vi "FindVideoDevices.vi"(8 "error in (no error)":errorcluster, 11 "Path to FFMPEG":path=path "C:/Program Files/FFMpeg/bin/ffmpeg.exe") -> (0 "error out":errorcluster, 3 "Video Devices":string[](array[string]))   [LabVIEW 2024]
uses:
  <userlib>/_OpenG.lib/array/array.llb/Conditional Auto-Indexing Tunnel (String)__ogtk.vi
  <vilib>/regexp/Match Regular Expression.xnode
  <userlib>/_OpenG.lib/string/string.llb/openg_string.lvlib
  <userlib>/_OpenG.lib/array/array.llb/openg_array.lvlib
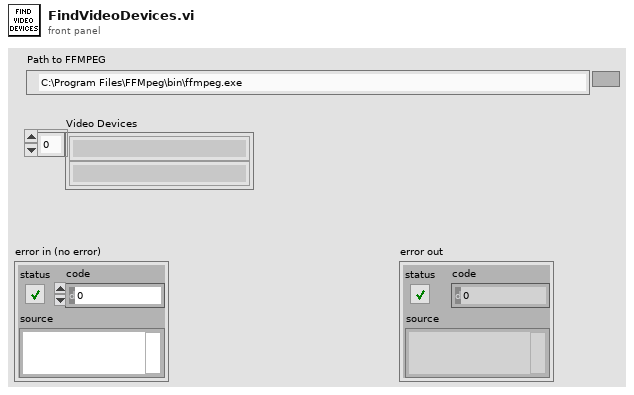
[diagram p1: front panel]
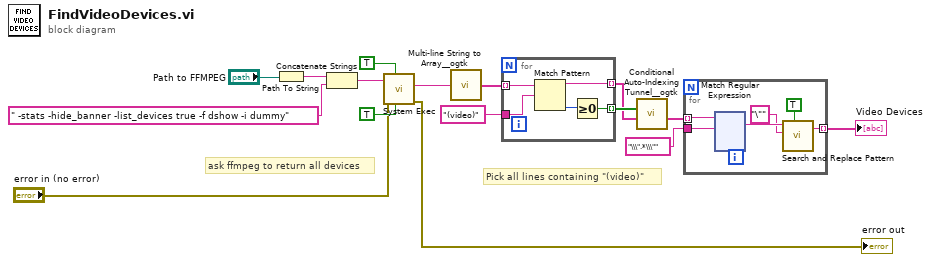
[diagram p0: block diagram]
diagram:
  # "ask ffmpeg to return all devices"
  # "Pick all lines containing \"(video)\""
  n1 = Path To String(path="Path to FFMPEG") -> (string=w15:string)
  n2 = Concatenate Strings(w15, " -stats -hide_banner -list_devices true -f dshow -i dummy") -> (w11:string)
  n3 = call <vilib>:"System Exec.vi"("run minimized? (F)"=TRUE, "wait until completion? (T)"=TRUE, "error in (no error)"="error in (no error)", "command line"=w11) -> ("error out"=→"error out":errorcluster, "standard error"=w10:string)  [unwired: 4 in, 2 out]
  n4 = call <userlib>:"Multi-line String to Array__ogtk.vi"("string"=w10) -> ("lines"=w9:string[])
  n5 = for {
    tunnel: w9 -> [w21] mode=indexing
    tunnel: "(video)" -> [w20]
    tunnel: [w19] -> w6 mode=indexing
    tunnel: [w17] -> w7 mode=indexing
    n6 = Match Pattern(string=w21, regular expression=w20) -> (before substring=w19:string, offset past match=w18:i32)  [unwired: 1 in, 2 out]
    n7 = Greater Or Equal To 0?(x=w18) -> (x >= 0?=w17:bool)
  }
  n8 = call-poly <userlib>:"Conditional Auto-Indexing Tunnel__ogtk.vi"("Array in"=w6, "Elements to keep"=w7) -> ("Filtered Array out"=w3:string[])  [unwired: 5 in]
  n9 = for {
    tunnel: w3 -> [w27] mode=indexing
    tunnel: "\\\".*\\\"" ("regular expression (\"\")") -> [w26]
    tunnel: [w23] -> w4 mode=indexing
    n10 = xnode "Match Regular Expression"("input string"=w27, "regular expression"=w26) -> ("whole match"=w24:string)  [unwired: 4 in, 4 out]
    n11 = call <vilib>:"Search and Replace Pattern.vi"("string"=w24, "regular expression (\"\")"="\"", "replace all? (F)"=TRUE) -> ("result string"=w23:string)  [unwired: 2 in, 1 out]
  }
  "Video Devices" <- w4
